vi "Elapsed Time.vi"(3 "error in (no error)":errorcluster, 4 "Title":string, 5 "Increment":dbl=0.01 min=0.01 max=1.0 step=0.01, 6 "Time Target (s)":dbl=1.0) -> (0 "error out":errorcluster)   [LabVIEW 2013]
uses:
  <vilib>/Utility/miscctls.llb/LVRangeTypeDef.ctl
panel:
  in  "Skip":bool
  out "Numeric":i32
  out "Time":dbl(slide) scale=0.0..120.0
  out "Elapsed Time (s)":dbl format="%#_3g"
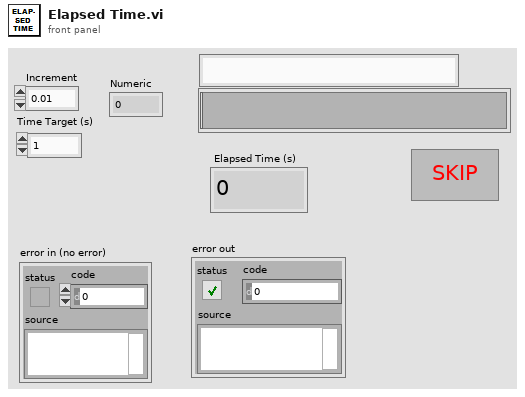
[diagram p1: front panel]
types:
  T1 = typedef "LVRangeTypeDef.ctl" = cluster{"Minimum":dbl, "Maximum":dbl, "Increment":dbl, "Minor Increment":dbl, "Start":dbl}
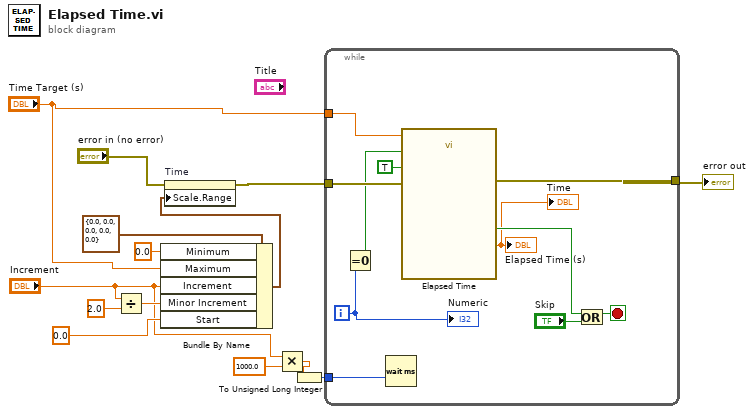
[diagram p0: block diagram]
diagram:
  n1 = Divide(x="Increment", y=2.0) -> (x/y=w9:dbl)
  n2 = Bundle By Name(cluster=T1 {"Minimum"=0.0, "Maximum"=0.0, "Increment"=0.0, "Minor Increment"=0.0, "Start"=0.0} ("Scale.Range"), "Minimum"=0.0, "Maximum"="Time Target (s)", "Increment"="Increment", "Minor Increment"=w9, "Start"=0.0 ("Increment")) -> (w6:T1)
  n3 = property on="Time" class="Slide (strict)"(error in="error in (no error)", "Scale.Range"=w6) -> (error out=w12:errorcluster)  [unwired: 1 in, 1 out]
  n4 = Multiply(x="Increment", y=1000.0) -> (x*y=w2:dbl)
  n5 = To Unsigned Long Integer(number=w2) -> (unsigned 32bit integer=w1:u32)
  n6 = while {
    tunnel: [w23] -> w14
    tunnel: w12 -> [w22]
    tunnel: "Time Target (s)" -> [w20]
    tunnel: w1 -> [w19]
    i -> [w16]
    stop <- w18 stop-if-true
    n7 = Equal To 0?(x=w16) -> (x = 0?=w15:bool)
    n8 = Wait (ms)(milliseconds to wait=w19) -> ()  [unwired: 1 out]
    n9 = call "Elapsed Time"("Time Target (s)"=w20, "Reset"=w15, "Auto Reset"=TRUE, "error in (no error)"=w22) -> ("Elapsed Time (s)"=→"Elapsed Time (s)" →"Time":dbl, "Time has Elapsed"=w25:bool, "error out"=w23:errorcluster)  [unwired: 8 in, 5 out]
    n10 = Or(x=w25, y="Skip") -> (x .or. y?=w18:bool)
    "Numeric" <- w16
  }
  "error out" <- w14
